vi "publish-battery-under-test.vi"() -> ()   [LabVIEW 2017, in "Library.lvlib"]
uses:
  Library.lvlib
  <vilib>/Skyline/Tag/Shared/typedefs/DataType.ctl
  <vilib>/Skyline/Message/HTTP Wrapper/Open (HTTP).vi
  <vilib>/Skyline/Tag/Wrapper/Wrapper HTTP_class/Open Tag HTTP.vi
  <vilib>/Skyline/Tag/Wrapper/Wrapper_class/Generate Tag Cluster (DBL) 2.vi
  <vilib>/Skyline/Tag/Wrapper/Wrapper_class/Close Tag (Multiple).vi
  <vilib>/Skyline/Message/HTTP Wrapper/NI Skyline Message HTTP.lvclass
  <vilib>/Skyline/Tag/Wrapper/Wrapper_class/NI Skyline Tag.lvclass
  <vilib>/Skyline/Tag/Shared/NI Skyline Tag.lvlib
  <vilib>/Skyline/Configuration/Configuration HTTP_class/NI Skyline Configuration HTTP.lvclass
  <vilib>/Skyline/Configuration/Configuration_class/NI Skyline Configuration.lvclass
  <vilib>/Skyline/Message/NI Skyline Message.lvclass
  <vilib>/Skyline/Tag/Wrapper/Wrapper HTTP_class/NI Skyline Tag HTTP.lvclass
  <vilib>/Skyline/Configuration/Configuration AMQP_class/Open Configuration AMQP.vi
  <vilib>/Skyline/Configuration/Configuration AMQP_class/NI Skyline Configuration AMQP.lvclass
  <vilib>/Skyline/Configuration/Configuration HTTP_class/Open Configuration HTTP.vi
panel:
  out "load-sweep":dbl[](graph) caption="Inner Temp (F)"
  in  "Stop":bool
  out "ramp-sweep":dbl[](graph) caption="Inner Temp (F)"
  # "Overview: Demonstrates the use of the Skyline Tag functions to write multiple tag values. Use tags to publish and monitor live measurement data.\n\nRequirements: LabVIEW NXG Web Module\n\nInstructions:\n1. Ensure the local SystemLink Server is running or you have access to SystemLink Cloud\n2. Determine if this example is connecting to data available on SystemLink Server or SystemLink Cloud and use the appropriate version of Open Configuration.vi \n3. Run this VI\n4. Monitor data published by this VI by running either ReadTags.gviweb or Main.gviweb in webvi-examples\\UtilizeSkylineDataServices\\UtilizeSkylineDataServices.lvproject"
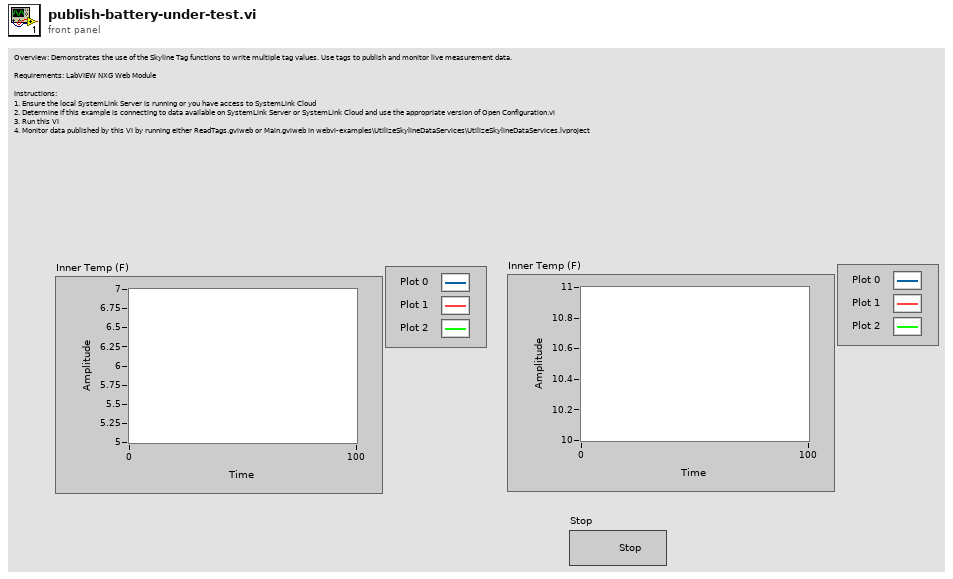
[diagram p1: front panel]
types:
  T1 = typedef "NI Skyline Tag.lvlib/DataType.ctl" = enum32{"Double", "Integer", "String"}
  T2 = typedef "NI Skyline Tag.lvclass/Tag Value Cluster Wrapper.ctl" = cluster{"Configuration":refnum<class "NI Skyline Configuration.lvclass">, "Tag Cluster":T3}
  T3 = typedef "NI Skyline Tag.lvlib/Tag Value Cluster.ctl" = cluster{"Path":string, "Data Type":T1, "Value":string, "Time Stamp":timestamp}
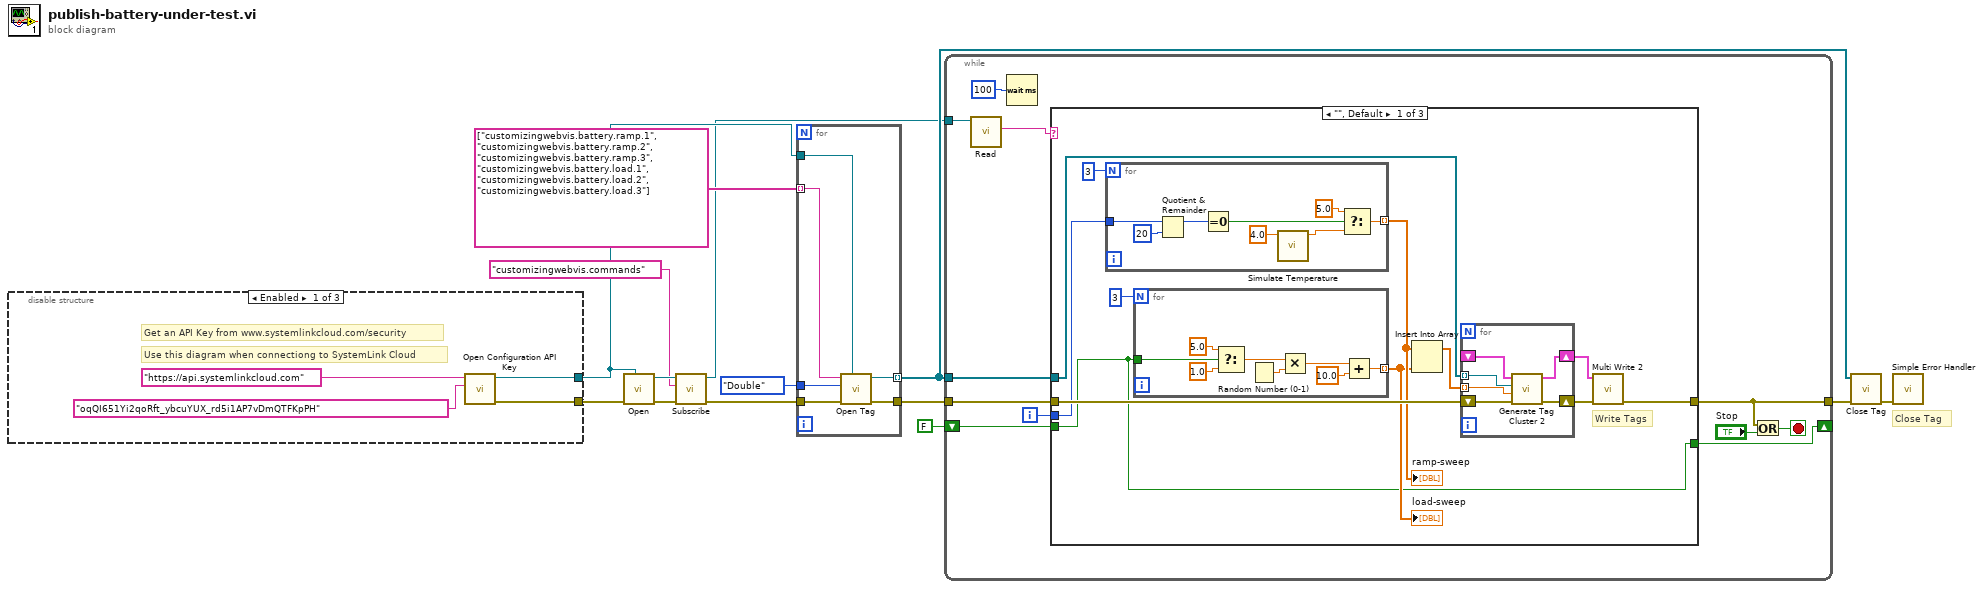
[diagram p0: block diagram]
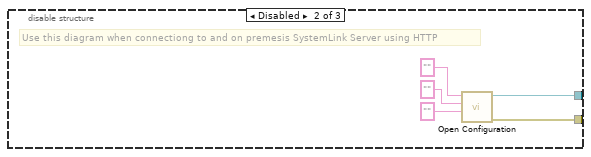
[diagram p2: hidden frame]
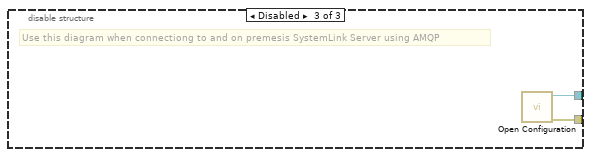
[diagram p3: hidden frame]
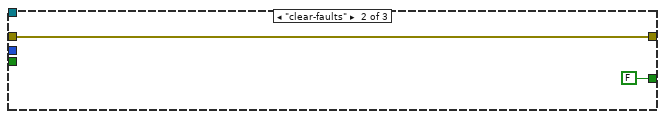
[diagram p4: hidden frame]
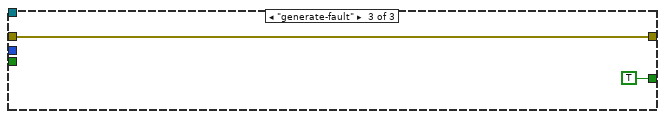
[diagram p5: hidden frame]
diagram:
  # "Close Tag"
  n1 = disable-structure shown="Enabled" {
    disable-tunnel: [w18 w19 w25] -> w8
    disable-tunnel: [w17 w23 w24] -> w7
    frame Enabled {
      # "Get an API Key from www.systemlinkcloud.com/security"
      # "Use this diagram when connectiong to SystemLink Cloud"
      n2 = call <vilib>:"Open Configuration API Key.vi"("api key"="oqQI651Yi2qoRft_ybcuYUX_rd5i1AP7vDmQTFKpPH", "server url"="https://api.systemlinkcloud.com") -> ("error out"=w17:errorcluster, "HTTP configuration out"=w18:refnum<class "NI Skyline Configuration HTTP.lvclass">)  [unwired: 8 in]
    }
    frame Disabled {
      # "Use this diagram when connectiong to and on premesis SystemLink Server using HTTP"
      n3 = call-poly <vilib>:"Open Configuration.vi"("password"="", "username"="", "server url"="") -> ("error out"=w23:errorcluster, "HTTP configuration out"=w19:refnum<class "NI Skyline Configuration HTTP.lvclass">)  [unwired: 7 in]
    }
    frame Disabled {
      # "Use this diagram when connectiong to and on premesis SystemLink Server using AMQP"
      n4 = call-poly <vilib>:"Open Configuration.vi"() -> ("error out"=w24:errorcluster, "AMQP configuration out"=w25:refnum<class "NI Skyline Configuration AMQP.lvclass">)  [unwired: 10 in]
    }
  }
  n5 = call-poly <vilib>:"Open.vi"("configuration"=w8, "error in (no error)"=w7) -> ("error out"=w6:errorcluster, "message http out"=w4:refnum<class "NI Skyline Message HTTP.lvclass">)  [unwired: 8 in]
  n6 = call-dynamic "Subscribe.vi"("error in (no error)"=w6, "topic"="customizingwebvis.commands", "message http"=w4) -> ("error out"=w5:errorcluster, "message http out"=w3:refnum<class "NI Skyline Message HTTP.lvclass">)  [unwired: 7 in]
  n7 = for {
    tunnel: w8 -> [w31]
    tunnel: w5 -> [w30]
    tunnel: DataType."Double" ("Data Type") -> [w29]
    tunnel: [w28] -> w11
    tunnel: string[] ["customizingwebvis.battery.ramp.1", "customizingwebvis.battery.ramp.2", "customizingwebvis.battery.ramp.3", "customizingwebvis.battery.load.1", "customizingwebvis.battery.load.2", "customizingwebvis.battery.load.3"] -> [w27] mode=indexing
    tunnel: [w26] -> w9 mode=indexing
    n8 = call-poly <vilib>:"Open Tag.vi"("configuration"=w31, "error in (no error)"=w30, "Data Type"=w29, "path"=w27) -> ("error out"=w28:errorcluster, "tag out"=w26:refnum<class "NI Skyline Tag.lvclass">)  [unwired: 6 in]
  }
  n9 = while {
    tunnel: [w40] -> w14
    tunnel: w11 -> [w39]
    tunnel: w9 -> [w38]
    tunnel: w3 -> [w35]
    shift-right: [w33] -> _
    shift-left: FALSE -> [w32]
    i -> [w37]
    stop <- w41 stop-if-true
    n10 = call-dynamic "Read.vi"("message http"=w35) -> ("topic"=w36:string)  [unwired: 6 in, 4 out]
    n11 = Wait (ms)(milliseconds to wait=u32 100) -> ()  [unwired: 1 out]
    n12 = case shown="\"\", Default" w36 {
      tunnel: [w54 w78 w79] -> w40
      tunnel: w39 -> [w52 w78 w79]
      tunnel: w38 -> [w51 _ _]
      tunnel: w37 -> [w49 _ _]
      tunnel: [w43 FALSE TRUE] -> w33
      tunnel: w32 -> [w43 _ _]
      frame "", Default {
        # "Write Tags"
        n13 = for {
          N: 3 -> [_]
          tunnel: [w65] -> w46 mode=indexing
          tunnel: w49 -> [w67]
          n14 = Quotient & Remainder(x=w67, y=20) -> (x-y*floor(x/y)=w69:i32)  [unwired: 1 out]
          n15 = Equal To 0?(x=w69) -> (x = 0?=w70:bool)
          n16 = call "Simulate Temperature.vi"("Starting Temp"=4.0) -> ("Temp (F)"=w66:dbl)  [unwired: 10 in]
          n17 = Select(t=5.0, s=w70, f=w66) -> (s? t:f=w65:dbl)
        }
        "ramp-sweep" <- w46
        n18 = for {
          N: 3 -> [_]
          tunnel: [w61] -> w44 mode=indexing
          tunnel: w43 -> [w60]
          n19 = Select(t=5.0, s=w60, f=1.0) -> (s? t:f=w57:dbl)
          n20 = Random Number (0-1)() -> (number: 0 to 1=w56:dbl)
          n21 = Multiply(x=w57, y=w56) -> (x*y=w55:dbl)
          n22 = Add(x=w55, y=10.0) -> (x+y=w61:dbl)
        }
        "load-sweep" <- w44
        n23 = Insert Into Array(array=w46, new element=w44) -> (w45:dbl[])  [unwired: 1 in]
        n24 = for {
          tunnel: w51 -> [w74] mode=indexing
          shift-right: [w76] -> w53
          shift-left: w52 -> [w75]
          tunnel: w45 -> [w73] mode=indexing
          shift-right: [w72] -> w50
          shift-left: _ -> [w71]
          n25 = call-poly <vilib>:"Generate Tag Cluster 2.vi"("error in (no error)"=w75, "value"=w73, "tag in"=w74, "tag clusters in"=w71) -> ("error out"=w76:errorcluster, "tag clusters out"=w72:T2[])  [unwired: 5 in, 1 out]
        }
        n26 = call <vilib>:"Multi Write 2.vi"("error in (no error)"=w53, "tag clusters"=w50) -> ("error out"=w54:errorcluster)  [unwired: 9 in]
      }
      frame "clear-faults" {
      }
      frame "generate-fault" {
      }
    }
    n27 = Or(x=w40, y="Stop") -> (x .or. y?=w41:bool)
  }
  n28 = call-poly <vilib>:"Close Tag.vi"("error in (no error)"=w14, "tags in"=w9) -> ("error out"=w13:errorcluster)  [unwired: 9 in]
  n29 = call <vilib>:"Simple Error Handler.vi"("error in (no error)"=w13) -> ()  [unwired: 4 in, 5 out]
